vi "flame2.vi"() -> ()   [LabVIEW 2019]
uses:
  <vilib>/MakerHub/LINX/Public/Peripherals/Digital/Digital Read 1 Chan.vi
  <vilib>/MakerHub/LINX/Public/Peripherals/Digital/Digital Write 1 Chan.vi
  <vilib>/MakerHub/LINX/Public/Peripherals/Digital/Digital Read N Chans.vi
  <vilib>/MakerHub/LINX/Public/Peripherals/Digital/Digital Write N Chans.vi
  <vilib>/MakerHub/LINX/Private/Local IO/LinxDigitalRead.vi
  <vilib>/MakerHub/LINX/Public/Utilities/Check Channel.vi
  <vilib>/MakerHub/LINX/Private/Local IO/LinxDigitalWrite.vi
  <vilib>/MakerHub/LINX/Public/Utilities/Open Serial.vi
  <vilib>/MakerHub/LINX/Private/Utilties/Generate Error.vi
  <vilib>/MakerHub/LINX/LMH-LINX.lvlib
panel:
  in  "Serial Port":refnum<visa-resource-name>="N/A"
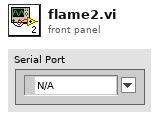
[diagram p1: front panel]
types:
  T1 = typedef "LMH-LINX.lvlib/LINX Ref.ctl" = cluster{"IO":T2, "Interface":T3, "LINX Device Config":T4}
  T2 = typedef "LMH-LINX.lvlib/Platform.ctl" = enum16{"Remote", "Local"}
  T3 = typedef "LMH-LINX.lvlib/Interface.ctl" = enum16{"Serial", "TCP"}
  T4 = typedef "LMH-LINX.lvlib/Device.lvlib/LINX Device Config.ctl" = cluster{"Interface":T3, "COM Port":refnum<visa-resource-name>, "TCP Configuration":T5, "Device Family":u8, "Device ID":u8, "Device Name":string, "TCP Ref":refnum<k5>, "Channels":T6}
  T5 = typedef "LMH-LINX.lvlib/Device.lvlib/TCP Config.ctl" = cluster{"IP Address":string, "Port":u16}
  T6 = typedef "LMH-LINX.lvlib/Channels.ctl" = cluster{"DI":u8[], "DO":u8[], "AI":u8[], "AO":u8[], "PWM":u8[], "QE":u8[], "UART":u8[], "I2C 2":u8[], "SPI":u8[], "CAN":u8[], "Servo":u8[], "AI Ref (V)":dbl, "AI Resolution (Bits)":u8, "AO Ref (V)":dbl, "AO Resolution (Bits)":u8}
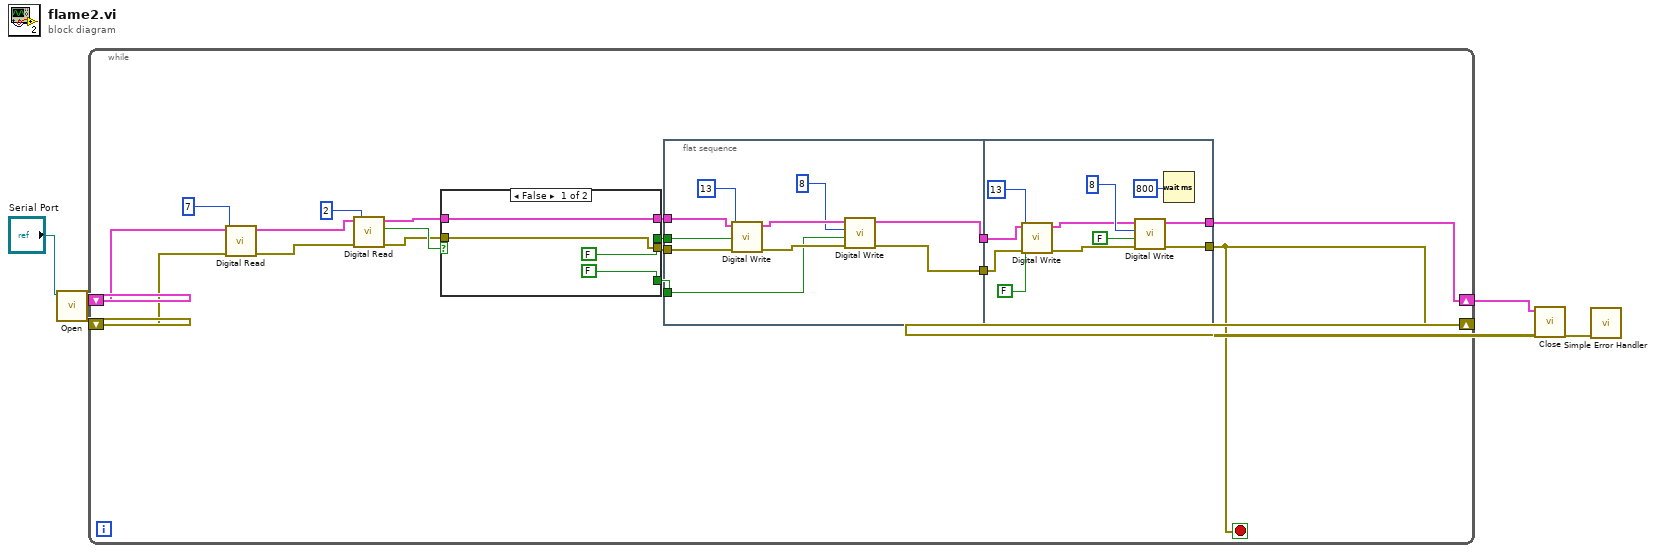
[diagram p0: block diagram]
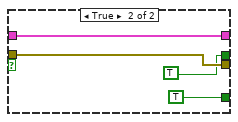
[diagram p2: hidden frame]
diagram:
  n1 = call-poly <vilib>:"Open.vi"("Serial Port"="Serial Port") -> ("Error Out"=w2:errorcluster, "LINX Resource"=w4:T1)  [unwired: 8 in, 1 out]
  n2 = while {
    shift-right: [w15] -> w1
    shift-left: w4 -> [w11]
    shift-right: [w7] -> w3
    shift-left: w2 -> [w12]
    stop <- w7 stop-if-true
    n3 = call-poly <vilib>:"Digital Read.vi"("Error In"=w12, "DI Channel"=u8 7, "LINX Resource"=w11) -> ("Error Out"=w8:errorcluster, "LINX Resource"=w9:T1)  [unwired: 6 in, 1 out]
    n4 = call-poly <vilib>:"Digital Read.vi"("Error In"=w8, "DI Channel"=u8 2, "LINX Resource"=w9) -> ("Error Out"=w21:errorcluster, "DI Value"=w22:bool, "LINX Resource"=w20:T1)  [unwired: 6 in]
    n5 = case shown="False" w22 {
      tunnel: [w47 w52] -> w18
      tunnel: w21 -> [w47 w52]
      tunnel: [w48 w51] -> w19
      tunnel: w20 -> [w48 w51]
      tunnel: [FALSE TRUE] -> w17
      tunnel: [FALSE TRUE] -> w16
      frame False {
      }
      frame True {
      }
    }
    n6 = flat-sequence {
      tunnel: w19 -> [w33]
      tunnel: [w31] -> w14
      tunnel: w18 -> [w30]
      tunnel: [w26] -> w13
      tunnel: w17 -> [w25]
      tunnel: w16 -> [w24]
      tunnel: w14 -> [w40]
      tunnel: w13 -> [w37]
      tunnel: [w39] -> w15
      tunnel: [w38] -> w7
      frame #0 {
        n7 = call-poly <vilib>:"Digital Write.vi"("Error In"=w30, "Output Value"=w25, "DO Channel"=u8 13, "LINX Resource"=w33) -> ("Error Out"=w29:errorcluster, "LINX Resource"=w32:T1)  [unwired: 6 in]
        n8 = call-poly <vilib>:"Digital Write.vi"("Error In"=w29, "Output Value"=w24, "DO Channel"=u8 8, "LINX Resource"=w32) -> ("Error Out"=w26:errorcluster, "LINX Resource"=w31:T1)  [unwired: 6 in]
      }
      frame #1 {
        n9 = call-poly <vilib>:"Digital Write.vi"("Error In"=w37, "Output Value"=FALSE, "DO Channel"=u8 13, "LINX Resource"=w40) -> ("Error Out"=w42:errorcluster, "LINX Resource"=w41:T1)  [unwired: 6 in]
        n10 = call-poly <vilib>:"Digital Write.vi"("Error In"=w42, "Output Value"=FALSE, "DO Channel"=u8 8, "LINX Resource"=w41) -> ("Error Out"=w38:errorcluster, "LINX Resource"=w39:T1)  [unwired: 6 in]
        n11 = Wait (ms)(milliseconds to wait=u32 800) -> ()  [unwired: 1 out]
      }
    }
  }
  n12 = call <vilib>:"Close.vi"("Error In"=w3, "LINX Resource"=w1) -> ("Error Out"=w5:errorcluster)  [unwired: 9 in]
  n13 = call <vilib>:"Simple Error Handler.vi"("error in (no error)"=w5) -> ()  [unwired: 4 in, 5 out]
